vi "Send_User_Event_Array.vi"(6 "priority (normal)":T1=enum."normal priority", 8 "error in (no error)":errorcluster, 9 "Data":variant[](array[variant]), 10 "Command":string[](array[string]), 11 "user event In":refnum<user-event>) -> (0 "error out":errorcluster, 3 "user event Out":refnum<user-event>)   [LabVIEW 2014, in "User_Event_Library.lvlib"]
uses:
  User_Event_Library.lvlib
  TypeDef.ctl
  <vilib>/event_ctls.llb/usereventprio.ctl
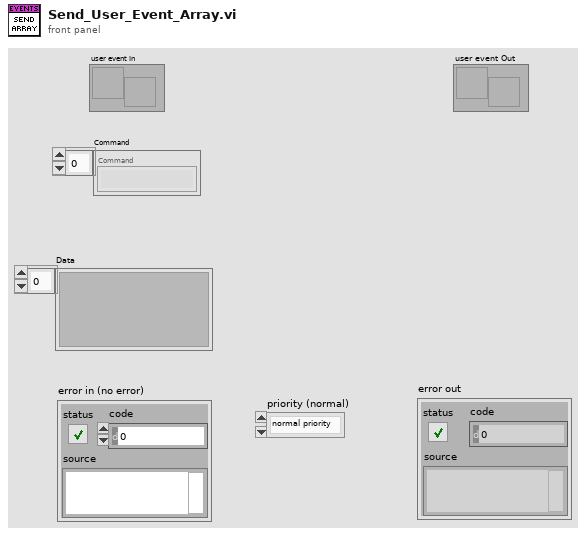
[diagram p1: front panel]
types:
  T1 = typedef "usereventprio.ctl" = enum32{"high priority", "normal priority"}
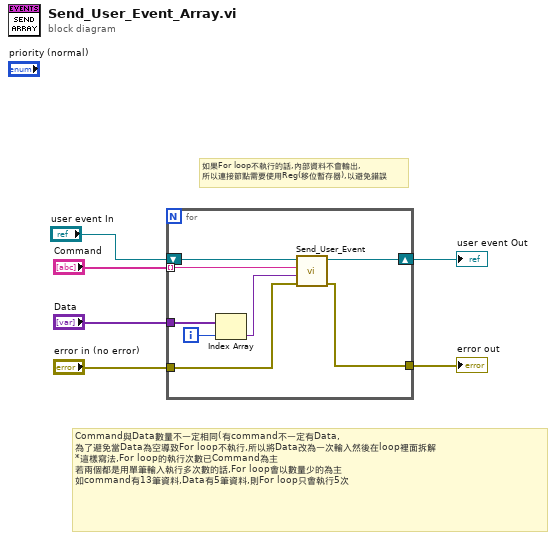
[diagram p0: block diagram]
diagram:
  # "Command與Data數量不一定相同(有command不一定有Data,\n為了避免當Data為空導致For loop不執行,所以將Data改為一次輸入然後在loop裡面拆解\n*這樣寫法,For loop的執行次數已Command為主\n若兩個都是用單筆輸入執行多次數的話,For loop會以數量少的為主\n如command有13筆資料,Data有5筆資料,則For loop只會執行5次"
  # "如果For loop不執行的話,內部資料不會輸出,\n所以連接節點需要使用Reg(移位暫存器),以避免錯誤"
  n1 = for {
    tunnel: [w12] -> w4
    shift-right: [w13] -> w5
    shift-left: "user event In" -> [w14]
    tunnel: "error in (no error)" -> [w11]
    tunnel: "Data" -> [w8]
    tunnel: "Command" -> [w7] mode=indexing
    i -> [w9]
    n2 = Index Array(array=w8, index=w9) -> (element=w10:variant)
    n3 = call "Send_User_Event.vi"("error in (no error)"=w11, "Data"=w10, "Command"=w7, "user event In"=w14) -> ("error out"=w12:errorcluster, "user event Out"=w13:refnum<user-event>)  [unwired: 6 in]
  }
  "error out" <- w4
  "user event Out" <- w5
